vi "MongoDB.CollectionReIndex.vi"(8 "error in (no error)":errorcluster, 11 "MongoDB.Collection in":refnum<class "MongoDB.Collection.lvclass">) -> (0 "error out":errorcluster, 3 "MongoDB.Collection out":refnum<class "MongoDB.Collection.lvclass">)   [LabVIEW 2014, in "MongoDB.Collection.lvclass"]
uses:
  MongoDB.Collection.lvclass
  MongoDB.Collection.lvclass/MongoDB.Collection.ctl
  C:/Users/Richard/Documents/GitHub/mongo-labview-driver/CSharp/bin/MongoDB.Driver.Legacy.dll
  CSharp/bin/MongoDB.Driver.Legacy.dll
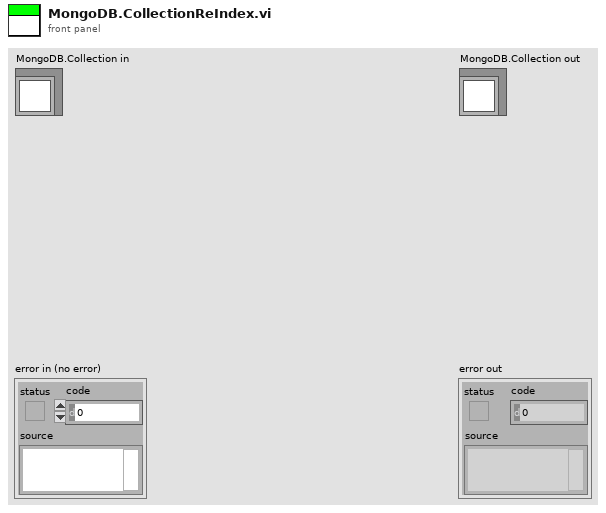
[diagram p1: front panel]
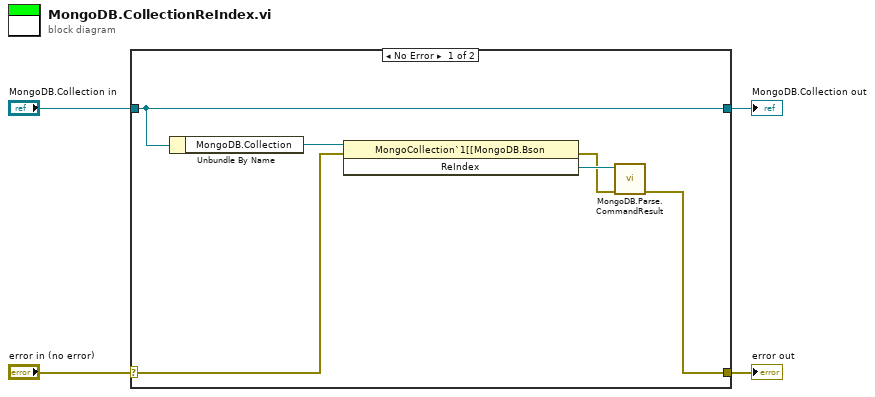
[diagram p0: block diagram]
diagram:
  n1 = case shown="No Error" "error in (no error)" {
    selector: "error in (no error)" -> [w8 w12]
    tunnel: [w5 w12] -> w3
    tunnel: [w10 w11] -> w1
    tunnel: "MongoDB.Collection in" -> [w10 w11]
    frame No Error {
      n2 = Unbundle By Name(w10) -> ("MongoDB.Collection"=w9:refnum<k24>)
      n3 = invoke class="MongoCollection`1[[MongoDB.Bson" method="ReIndex"(reference=w9, error in=w8) -> (error out=w6:errorcluster, "ReIndex"=w7:refnum<k24>)  [unwired: 1 in, 1 out]
      n4 = call "MongoDB.Parse.CommandResult.vi"("error in (no error)"=w6, "MongoDB.Command.Result"=w7) -> ("error out"=w5:errorcluster)  [unwired: 9 in]
    }
    frame Error {
    }
  }
  "error out" <- w3
  "MongoDB.Collection out" <- w1
